vi "Autonomous Independent (3).vi"() -> ()   [LabVIEW 2016]
doc: "This VI is called when autonomous begins, and will automatically be terminated when autonomous ends. You can carry out timed or sensor driven robot movement independently without needing to return to the caller."
uses:
  <vilib>/Rock Robotics/WPI/Solenoid/WPI_SolenoidValue.ctl
  <vilib>/Rock Robotics/Network Tables/NT Read String.vi
  <vilib>/Rock Robotics/WPI/Solenoid/WPI_SolenoidSetEnum.vi
panel:
  in  "Target Angle":dbl
  out "Refnum's Out":T1
  in  "Target Distance":dbl=15.0 format="%#_13g"
  out "Error Out":errorcluster
  in  "Error In":errorcluster
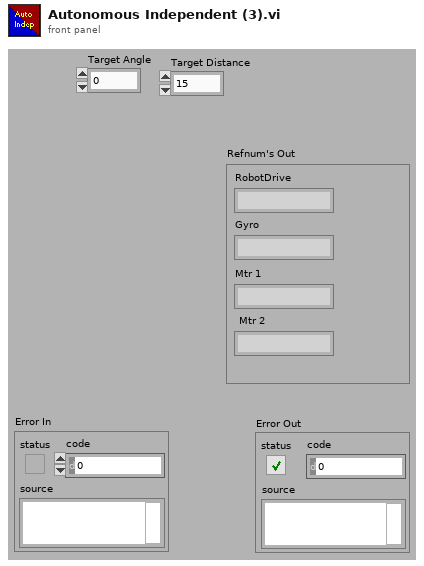
[diagram p1: front panel]
types:
  T1 = cluster{"RobotDrive":string, "Gyro":string, "Mtr 1":string, "Mtr 2":string}
  T2 = typedef "WPI_SolenoidValue.ctl" = enum16{"Off", "On", "Forward", "Reverse"}
  T3 = cluster{"Gyro":string, "Mtr 1":string, "Mtr 2":string}
  T4 = typedef "WPI_MotorControlDeviceRef.ctl" = cluster{"DeviceStatus":errorcluster, "Type":T5, "PWM":cluster{"PWM Channel":T6, "DeadBand":T7}, "CAN":cluster{"Device Number":u8, "SetOutput VI Ref":variant, "GetOutput VI Ref":variant, "Enable VI Ref":variant, "Disable VI Ref":variant, "Data":variant}, "Invert":bool}
  T5 = typedef "WPI_MotorControlType.ctl" = enum16{"PWM", "CAN"}
  T6 = typedef "FPGA_DIOPWMChannel.ctl" = enum8{"PWM 0", "PWM 1", "PWM 2", "PWM 3", "PWM 4", "PWM 5", "PWM 6", "PWM 7", "PWM 8", "PWM 9", "PWM MXP 0", "PWM MXP 1", "PWM MXP 2", "PWM MXP 3", "PWM MXP 4", "PWM MXP 5", "PWM MXP 6", "PWM MXP 7", "PWM MXP 8", "PWM MXP 9", "Invalid"}
  T7 = typedef "WPI_PWMDeadband.ctl" = cluster{"Name":string, "maxPositivePwm":i32, "minPositivePwm":i32, "centerPwm":i32, "maxNegativePwm":i32, "minNegativePwm":i32, "angularRange":u16}
  T8 = typedef "WPI_GyroDevRef.ctl" = cluster{"DevStatus":errorcluster, "Analog Channel":T9, "Offset":dbl, "Gain (VoltsPerDegree/Second)":dbl, "Gyro Type":enum16{"Analog", "XRS450"}, "Handle":i32, "SPI Bus":T10, "Device Found":bool, "Sample Rate":dbl, "Calibrate On Open":bool}
  T9 = typedef "FPGA_AIChannel.ctl" = enum8{"AI 0", "AI 1", "AI 2", "AI 3", "AI MXP 0", "AI MXP 1", "AI MXP 2", "AI MXP 3", "Invalid"}
  T10 = typedef "spi_bus.ctl" = enum16{"SPI On-Board, CS0", "SPI On-Board, CS1", "SPI On-Board, CS2", "SPI On-Board, CS3", "SPI MXP", "Invalid"}
  T11 = typedef "WPI_SolenoidDevRef.ctl" = cluster{"DevStatus":errorcluster, "Pneumatics Control Module":u8, "Forward Solenoid Channel":T12, "Reverse Solenoid Channel":T12}
  T12 = typedef "WPI_SolenoidChannel.ctl" = enum8{"Solenoid 0", "Solenoid 1", "Solenoid 2", "Solenoid 3", "Solenoid 4", "Solenoid 5", "Solenoid 6", "Solenoid 7", "Invalid"}
  T13 = typedef "WPI_DriverStationAllianceInfo.ctl" = enum16{"Red", "Blue", "Invalid"}
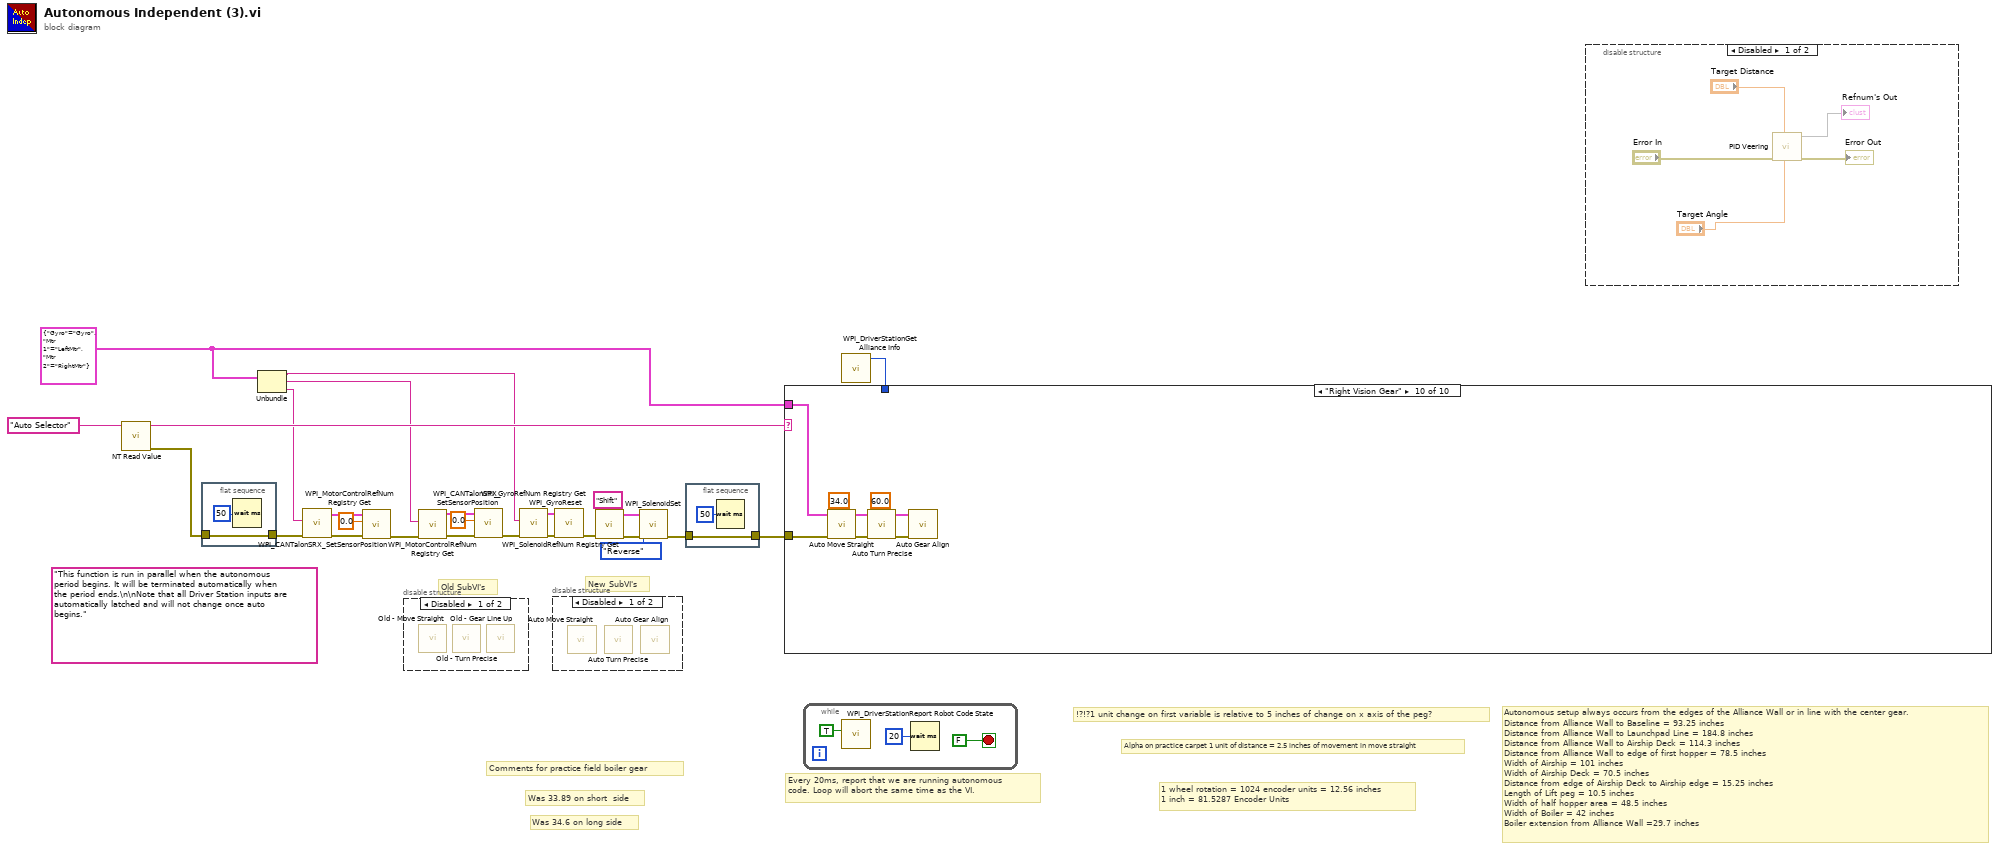
[diagram p0: block diagram]
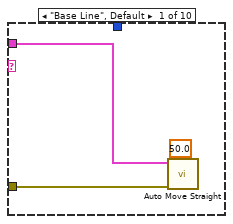
[diagram p3: hidden frame]
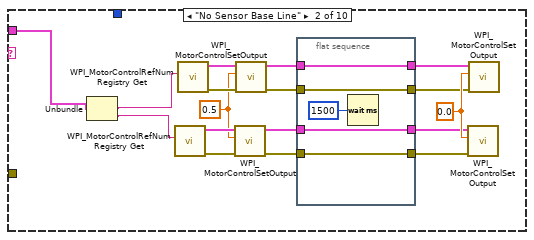
[diagram p4: hidden frame]
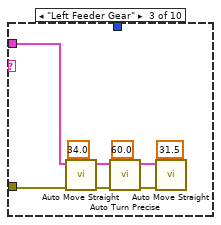
[diagram p5: hidden frame]
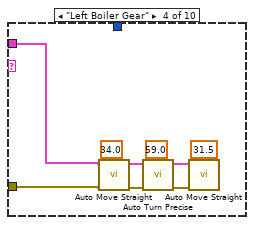
[diagram p6: hidden frame]
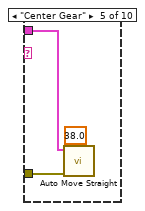
[diagram p7: hidden frame]
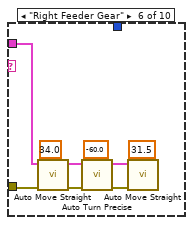
[diagram p8: hidden frame]
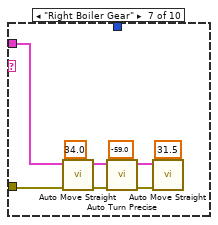
[diagram p9: hidden frame]
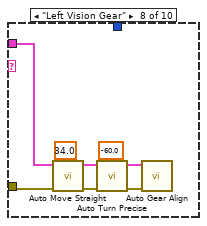
[diagram p10: hidden frame]
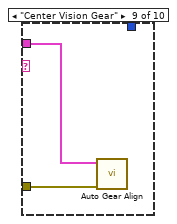
[diagram p11: hidden frame]
diagram:
  w4 = T3 {"Gyro"="Gyro", "Mtr 1"="LeftMtr", "Mtr 2"="RightMtr"} ("Refnum's")
  (unwired) "This function is run in parallel when the autonomous period begins. It will be terminated automatically when the period ends.\n\nNote that all Driver Station inputs are automatically latched and will not change once auto begins."
  # "Comments for practice field boiler gear"
  # "Was 34.6 on long side"
  # "Was 33.89 on short  side"
  # "!?!?1 unit change on first variable is relative to 5 inches of change on x axis of the peg?"
  # "Alpha on practice carpet 1 unit of distance = 2.5 inches of movement in move straight"
  # "New SubVI's"
  # "Old SubVI's"
  # "Autonomous setup always occurs from the edges of the Alliance Wall or in line with the center gear.\nDistance from Alliance Wall to Baseline = 93.25 inches\nDistance from Alliance Wall to Launchpad Line = 184.8 inches\nDistance from Alliance Wall to Airship Deck = 114.3 inches\nDistance from Alliance Wall to edge of first hopper = 78.5 inches\nWidth of Airship = 101 inches\nWidth of Airship Deck = 70.5 inches\nDistance from edge of Airship Deck to Airship edge = 15.25 inches\nLength of Lift peg = 10.5 inches\nWidth of half hopper area = 48.5 inches\nWidth of Boiler = 42 inches\nBoiler extension from Alliance Wall =29.7 inches"
  # "1 wheel rotation = 1024 encoder units = 12.56 inches\n1 inch = 81.5287 Encoder Units"
  # "Every 20ms, report that we are running autonomous\ncode. Loop will abort the same time as the VI."
  n1 = call-poly <vilib>:"NT Read Value.vi"("Name"="Auto Selector") -> ("error out"=w24:errorcluster, "String"=w25:string)  [unwired: 9 in]
  n2 = flat-sequence {
    tunnel: [w27] -> w10
    tunnel: w24 -> [w27]
    frame #0 {
      n3 = Wait (ms)(milliseconds to wait=u32 50) -> ()  [unwired: 1 out]
    }
  }
  n4 = Unbundle(w4) -> ("Gyro"=w3:string, "Mtr 1"=w2:string, "Mtr 2"=w1:string)
  n5 = call <vilib>:"WPI_MotorControlRefNum Registry Get.vi"("error in (no error)"=w10, "refnum name"=w1) -> ("error out"=w12:errorcluster, "MotorControlDevRef"=w13:T4)  [unwired: 8 in]
  n6 = call <vilib>:"WPI_CANTalonSRX_SetSensorPosition.vi"("error in (no error)"=w12, "New Sensor Position"=0.0, "CAN Talon SRX Ref"=w13) -> ("error out"=w9:errorcluster)  [unwired: 7 in, 1 out]
  n7 = disable-structure shown="Disabled" {
    frame Disabled {
      n8 = call "Old - Move Straight.vi"() -> ()  [unwired: 11 in, 1 out]
      n9 = call "Old - Turn Precise.vi"() -> ()  [unwired: 11 in, 1 out]
      n10 = call "Old - Gear Line Up.vi"() -> ()  [unwired: 11 in, 1 out]
    }
    frame Enabled {
    }
  }
  n11 = call <vilib>:"WPI_MotorControlRefNum Registry Get.vi"("error in (no error)"=w9, "refnum name"=w2) -> ("error out"=w15:errorcluster, "MotorControlDevRef"=w16:T4)  [unwired: 8 in]
  n12 = call <vilib>:"WPI_CANTalonSRX_SetSensorPosition.vi"("error in (no error)"=w15, "New Sensor Position"=0.0, "CAN Talon SRX Ref"=w16) -> ("error out"=w8:errorcluster)  [unwired: 7 in, 1 out]
  n13 = call <vilib>:"WPI_GyroRefNum Registry Get.vi"("error in (no error)"=w8, "refnum name"=w3) -> ("error out"=w23:errorcluster, "GyroDevRef"=w22:T8)  [unwired: 8 in]
  n14 = disable-structure shown="Disabled" {
    frame Disabled {
      n15 = call "Auto Move Straight.vi"() -> ()  [unwired: 10 in, 2 out]
      n16 = call "Auto Turn Precise.vi"() -> ()  [unwired: 10 in, 2 out]
      n17 = call "Auto Gear Align.vi"() -> ()  [unwired: 10 in, 2 out]
    }
    frame Enabled {
    }
  }
  n18 = call <vilib>:"WPI_GyroReset.vi"("error in"=w23, "GyroDevRef"=w22) -> ("error out"=w17:errorcluster)  [unwired: 8 in, 1 out]
  n19 = call <vilib>:"WPI_SolenoidRefNum Registry Get.vi"("error in (no error)"=w17, "refnum name"="Shift") -> ("error out"=w21:errorcluster, "SolenoidDevRef"=w20:T11)  [unwired: 8 in]
  n20 = call-poly <vilib>:"WPI_SolenoidSet.vi"("error in (no error)"=w21, "Value"=WPI_SolenoidValue."Reverse", "SolenoidDevRef"=w20) -> ("error out"=w5:errorcluster)  [unwired: 7 in, 1 out]
  n21 = flat-sequence {
    tunnel: [w29] -> w6
    tunnel: w5 -> [w29]
    frame #0 {
      n22 = Wait (ms)(milliseconds to wait=u32 50) -> ()  [unwired: 1 out]
    }
  }
  n23 = while {
    stop <- FALSE stop-if-true
    n24 = call <vilib>:"WPI_DriverStationReport Robot Code State.vi"("Autonomous"=TRUE) -> ()  [unwired: 10 in, 1 out]
    n25 = Wait (ms)(milliseconds to wait=u32 20) -> ()  [unwired: 1 out]
  }
  n26 = call <vilib>:"WPI_DriverStationGet Alliance Info.vi"() -> ("Alliance"=w7:T13)  [unwired: 10 in, 1 out]
  n27 = case shown="\"Right Vision Gear\"" w25 {
    tunnel: w4 -> [w36 w39 w62 w68 w78 w80 w89 w98 w106 w108]
    tunnel: w6 -> [w35 _ w63 w69 w79 w81 w90 w99 w107 w109]
    tunnel: w7 -> [_ _ _ _ _ _ _ _ _ _]
    frame "Base Line", Default {
      n28 = call "Auto Move Straight.vi"("Target Distance"=50.0, "Error In"=w35, "Refnum's In"=w36) -> ()  [unwired: 7 in, 2 out]
    }
    frame "No Sensor Base Line" {
      w48 = 0.0 ("Output")
      w49 = 0.5 ("Output")
      n29 = Unbundle(w39) -> ("Mtr 1"=w38:string, "Mtr 2"=w37:string)  [unwired: 1 out]
      n30 = call <vilib>:"WPI_MotorControlRefNum Registry Get.vi"("refnum name"=w37) -> ("error out"=w52:errorcluster, "MotorControlDevRef"=w53:T4)  [unwired: 9 in]
      n31 = call <vilib>:"WPI_MotorControlRefNum Registry Get.vi"("refnum name"=w38) -> ("error out"=w51:errorcluster, "MotorControlDevRef"=w50:T4)  [unwired: 9 in]
      n32 = call <vilib>:"WPI_MotorControlSetOutput.vi"("error in (no error)"=w52, "Output"=w49, "MotorControlDevRef"=w53) -> ("error out"=w42:errorcluster, "MotorControlDevRef"=w46:T4)  [unwired: 6 in, 1 out]
      n33 = call <vilib>:"WPI_MotorControlSetOutput.vi"("error in (no error)"=w51, "Output"=w49, "MotorControlDevRef"=w50) -> ("error out"=w41:errorcluster, "MotorControlDevRef"=w45:T4)  [unwired: 6 in, 1 out]
      n34 = flat-sequence {
        tunnel: [w57] -> w47
        tunnel: w46 -> [w57]
        tunnel: w45 -> [w56]
        tunnel: [w56] -> w44
        tunnel: [w55] -> w43
        tunnel: w42 -> [w55]
        tunnel: w41 -> [w54]
        tunnel: [w54] -> w40
        frame #0 {
          n35 = Wait (ms)(milliseconds to wait=u32 1500) -> ()  [unwired: 1 out]
        }
      }
      n36 = call <vilib>:"WPI_MotorControlSetOutput.vi"("error in (no error)"=w43, "Output"=w48, "MotorControlDevRef"=w47) -> ()  [unwired: 6 in, 3 out]
      n37 = call <vilib>:"WPI_MotorControlSetOutput.vi"("error in (no error)"=w40, "Output"=w48, "MotorControlDevRef"=w44) -> ()  [unwired: 6 in, 3 out]
    }
    frame "Left Feeder Gear" {
      n38 = call "Auto Move Straight.vi"("Target Distance"=34.0, "Error In"=w63, "Refnum's In"=w62) -> ("Error Out"=w67:errorcluster, "Refnum's Out"=w66:T3)  [unwired: 7 in]
      n39 = call "Auto Turn Precise.vi"("Target Distance"=60.0, "Error In"=w67, "Refnum's In"=w66) -> ("Error Out"=w65:errorcluster, "Refnum's Out"=w64:T3)  [unwired: 7 in]
      n40 = call "Auto Move Straight.vi"("Target Distance"=31.5, "Error In"=w65, "Refnum's In"=w64) -> ()  [unwired: 7 in, 2 out]
    }
    frame "Left Boiler Gear" {
      n41 = call "Auto Move Straight.vi"("Target Distance"=34.0, "Error In"=w69, "Refnum's In"=w68) -> ("Error Out"=w76:errorcluster, "Refnum's Out"=w75:T3)  [unwired: 7 in]
      n42 = call "Auto Turn Precise.vi"("Target Distance"=59.0, "Error In"=w76, "Refnum's In"=w75) -> ("Error Out"=w74:errorcluster, "Refnum's Out"=w73:T3)  [unwired: 7 in]
      n43 = call "Auto Move Straight.vi"("Target Distance"=31.5, "Error In"=w74, "Refnum's In"=w73) -> ()  [unwired: 7 in, 2 out]
    }
    frame "Center Gear" {
      n44 = call "Auto Move Straight.vi"("Target Distance"=38.0, "Error In"=w79, "Refnum's In"=w78) -> ()  [unwired: 7 in, 2 out]
    }
    frame "Right Feeder Gear" {
      n45 = call "Auto Move Straight.vi"("Target Distance"=34.0, "Error In"=w81, "Refnum's In"=w80) -> ("Error Out"=w82:errorcluster, "Refnum's Out"=w83:T3)  [unwired: 7 in]
      n46 = call "Auto Turn Precise.vi"("Target Distance"=-60.0, "Error In"=w82, "Refnum's In"=w83) -> ("Error Out"=w84:errorcluster, "Refnum's Out"=w85:T3)  [unwired: 7 in]
      n47 = call "Auto Move Straight.vi"("Target Distance"=31.5, "Error In"=w84, "Refnum's In"=w85) -> ()  [unwired: 7 in, 2 out]
    }
    frame "Right Boiler Gear" {
      n48 = call "Auto Move Straight.vi"("Target Distance"=34.0, "Error In"=w90, "Refnum's In"=w89) -> ("Error Out"=w91:errorcluster, "Refnum's Out"=w92:T3)  [unwired: 7 in]
      n49 = call "Auto Turn Precise.vi"("Target Distance"=-59.0, "Error In"=w91, "Refnum's In"=w92) -> ("Error Out"=w93:errorcluster, "Refnum's Out"=w94:T3)  [unwired: 7 in]
      n50 = call "Auto Move Straight.vi"("Target Distance"=31.5, "Error In"=w93, "Refnum's In"=w94) -> ()  [unwired: 7 in, 2 out]
    }
    frame "Left Vision Gear" {
      n51 = call "Auto Move Straight.vi"("Target Distance"=34.0, "Error In"=w99, "Refnum's In"=w98) -> ("Error Out"=w105:errorcluster, "Refnum's Out"=w104:T3)  [unwired: 7 in]
      n52 = call "Auto Turn Precise.vi"("Target Distance"=-60.0, "Error In"=w105, "Refnum's In"=w104) -> ("Error Out"=w101:errorcluster, "Refnum's Out"=w100:T3)  [unwired: 7 in]
      n53 = call "Auto Gear Align.vi"("Error In"=w101, "Refnum's In"=w100) -> ()  [unwired: 8 in, 2 out]
    }
    frame "Center Vision Gear" {
      n54 = call "Auto Gear Align.vi"("Error In"=w107, "Refnum's In"=w106) -> ()  [unwired: 8 in, 2 out]
    }
    frame "Right Vision Gear" {
      n55 = call "Auto Move Straight.vi"("Target Distance"=34.0, "Error In"=w109, "Refnum's In"=w108) -> ("Error Out"=w110:errorcluster, "Refnum's Out"=w111:T3)  [unwired: 7 in]
      n56 = call "Auto Turn Precise.vi"("Target Distance"=60.0, "Error In"=w110, "Refnum's In"=w111) -> ("Error Out"=w114:errorcluster, "Refnum's Out"=w115:T3)  [unwired: 7 in]
      n57 = call "Auto Gear Align.vi"("Error In"=w114, "Refnum's In"=w115) -> ()  [unwired: 8 in, 2 out]
    }
  }
  n58 = disable-structure shown="Disabled" {
    frame Disabled {
      n59 = call "PID Veering.vi"("Error"="Target Angle", "Current Distance"="Target Distance", "error in (no error)"="Error In") -> ("error out"=→"Error Out":errorcluster, 3:→"Refnum's Out")  [unwired: 7 in]
    }
    frame Enabled {
    }
  }
